vi "push_2_grab+normalize&cut.vi"() -> (11 "Array":u8[][](array[numeric]))   [LabVIEW 2015]
uses:
  <vilib>/userdefined/High Color/IMAQdx.ctl
  <vilib>/vision/driver/NI_Vision_Acquisition_Software.lvlib
panel:
  out "Numeric":i32
  out "Matches (pixel)":T1(array[cluster])
  in  "Path to template":path
  out "output 1":i32
  in  "Path 7":path
  in  "stop 2":bool
  in  "Boolean 2":bool
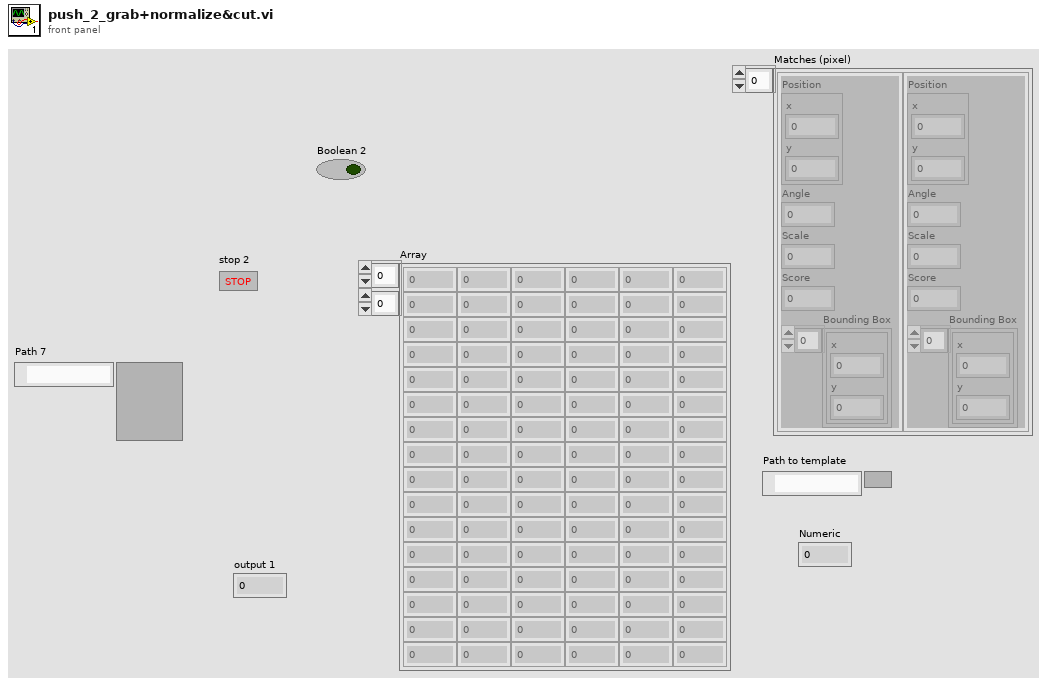
[diagram p1: front panel]
types:
  T1 = cluster{"Position":cluster{"x":sgl, "y":sgl}, "Angle":sgl, "Scale":sgl, "Score":sgl, "Bounding Box":cluster{"x":sgl, "y":sgl}[]}[]
  T2 = typedef "IMAQdx.ctl" = refnum<k21>
  T3 = enum16{"open", "replace", "create", "open or create", "replace or create", "replace or create with confirmation"}
  T4 = cluster{"Position":cluster{"x":sgl, "y":sgl}, "Angle":sgl, "Scale":sgl, "Score":sgl, "Bounding Box":cluster{"x":sgl, "y":sgl}[]}
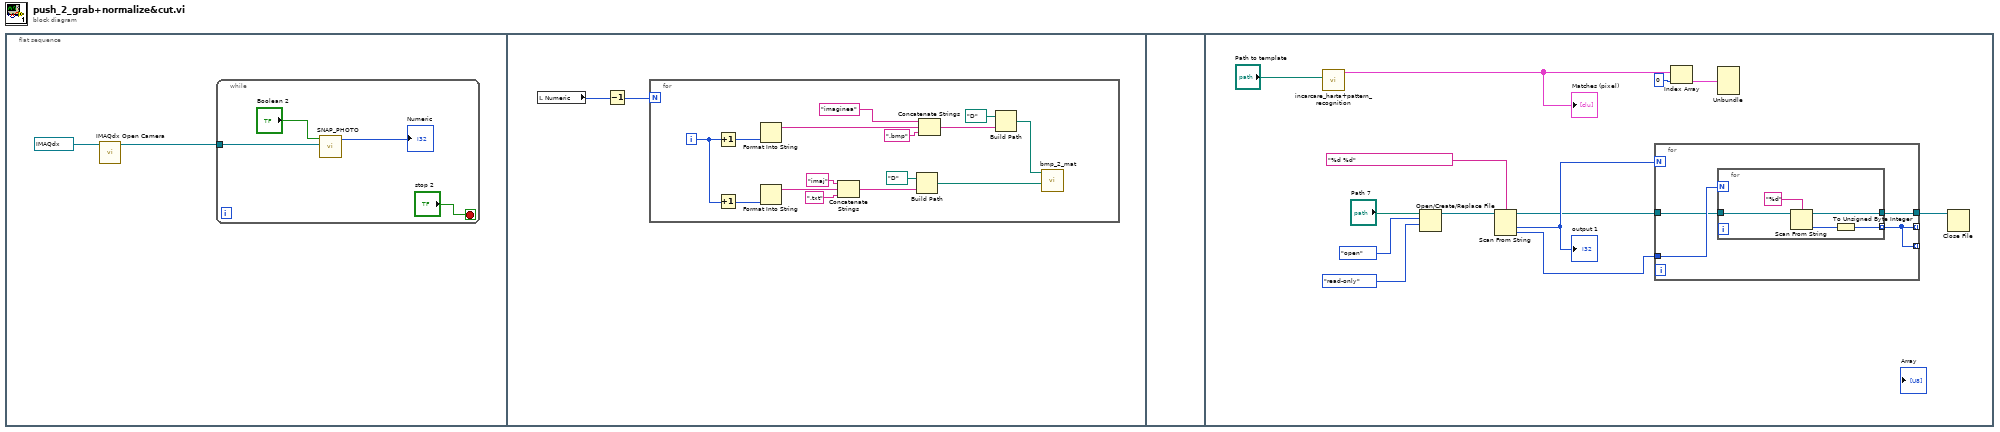
[diagram p0: block diagram]
diagram:
  n1 = flat-sequence {
    frame #0 {
      n2 = call <vilib>:"IMAQdx Open Camera.vi"("Session In"=T2 "cam0") -> ("Session Out"=w1:T2)  [unwired: 9 in, 1 out]
      n3 = while {
        tunnel: w1 -> [w5]
        stop <- "stop 2" stop-if-true
        n4 = call "SNAP_PHOTO.vi"("Session Out"=w5, "Boolean"="Boolean 2") -> ("Numeric 2"=→"Numeric":i32)  [unwired: 9 in]
      }
    }
    frame #1 {
      n5 = local read "Numeric"() -> (w7:i32)
      n6 = Decrement(x=w7) -> (x-1=w8:i32)
      n7 = for {
        N: w8 -> [_]
        i -> [w13]
        n8 = Increment(x=w13) -> (x+1=w10:i32)
        n9 = Increment(x=w13) -> (x+1=w9:i32)
        n10 = Format Into String(w10) -> (resulting string=w22:string)  [unwired: 3 in, 1 out]
        n11 = Format Into String(w9) -> (resulting string=w16:string)  [unwired: 3 in, 1 out]
        n12 = Concatenate Strings("imaj" ("string"), w16, ".txt" ("string")) -> (w12:string)
        n13 = Build Path(base path=path "D:/", name or relative path=w12) -> (appended path=w11:path)
        n14 = Concatenate Strings("imaginea" ("string"), w22, ".bmp" ("string")) -> (w19:string)
        n15 = Build Path(base path=path "D:/", name or relative path=w19) -> (appended path=w18:path)
        n16 = call "bmp_2_mat.vi"("Destinatia1"=w11, "Imaginea1"=w18) -> ()  [unwired: 10 in]
      }
    }
    frame #2 {
    }
    frame #3 {
      n17 = call "incarcare_harta+pattern_recognition.vi"("Find"="Path to template") -> ("Matches (pixel)"=w26:T1)  [unwired: 10 in]
      "Matches (pixel)" <- w26
      n18 = Open/Create/Replace File(file path (use dialog)="Path 7", operation (0:open)=T3."open", access (0:read/write)=enum16{"read/write", "read-only", "write-only"}."read-only") -> (refnum out=w33:refnum<file>)  [unwired: 3 in, 2 out]
      n19 = Scan From String("%d %d" ("format string"), w33) -> (w29:refnum<file>, output 1=w31:i32, output 2=w30:i32)  [unwired: 3 in, 1 out]
      "output 1" <- w31
      n20 = for {
        N: w31 -> [_]
        tunnel: w30 -> [w40]
        tunnel: w29 -> [w39]
        tunnel: [w37] -> _ mode=indexing
        tunnel: [w38] -> w28
        tunnel: [w37] -> _ mode=indexing
        n21 = for {
          N: w40 -> [_]
          tunnel: w39 -> [w45]
          tunnel: [w41] -> w37 mode=indexing
          tunnel: [w43] -> w38
          n22 = Scan From String("%d" ("format string"), w45) -> (w43:refnum<file>, output 1=w42:i32)  [unwired: 2 in, 1 out]
          n23 = To Unsigned Byte Integer(number=w42) -> (unsigned 8bit integer=w41:u8)
        }
      }
      n24 = Index Array(array=w26, index=0) -> (element=w24:T4)
      n25 = Unbundle(w24) -> ()  [unwired: 5 out]
      n26 = Close File(refnum=w28) -> ()  [unwired: 1 in, 2 out]
    }
  }
